vi "Init_Fingers.vi"(8 "error in (no error)":errorcluster) -> (0 "error out":errorcluster)   [LabVIEW 2019, in "Kinova MICO² USB.lvlib"]
uses:
  <vilib>/Utility/error.llb/Error Cluster From Error Code.vi
  <vilib>/ErrorRing/Error Ring.xnode
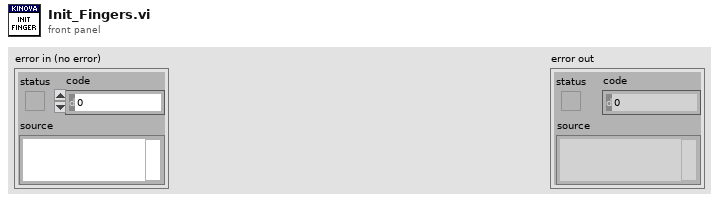
[diagram p1: front panel]
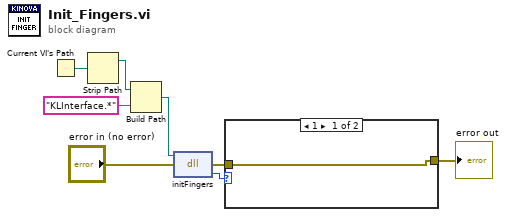
[diagram p0: block diagram]
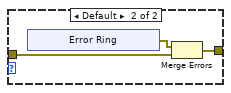
[diagram p2: hidden frame]
diagram:
  n1 = Current VI's Path() -> (path=w6:path)
  n2 = Strip Path(path=w6) -> (stripped path=w5:path)  [unwired: 1 out]
  n3 = Build Path(base path=w5, name or relative path="KLInterface.*") -> (appended path=w1:path)
  n4 = dll-call lib="C:/Users/mcjssdcc/source/repos/Kinova Labview Interface/Debug/KLInterface.dll" fn="initFingers"(path in=w1, error in="error in (no error)") -> (error out=w4:errorcluster, "return type"=w3:i32)  [unwired: 1 in, 1 out]
  n5 = case shown="1" w3 {
    tunnel: [w9 w11] -> w2
    tunnel: w4 -> [w9 w10]
    frame 1 {
    }
    frame Default {
      n6 = xnode "Error Ring"() -> ("error out"=w12:errorcluster)
      n7 = Merge Errors(w12, w10) -> (w11:errorcluster)
    }
  }
  "error out" <- w2
